vi "Henries Converter.vi"(1 "L in":dbl, 2 "L Units":enum16{"H", "mH", "µH", "nH", "pH"}(ring)) -> (0 "L out":dbl)   [LabVIEW 2013]
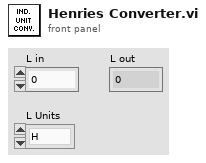
[diagram p1: front panel]
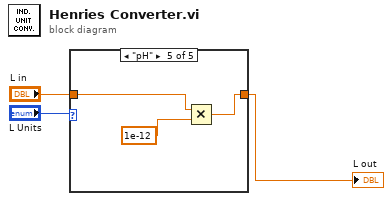
[diagram p0: block diagram]
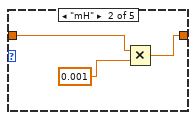
[diagram p3: hidden frame]
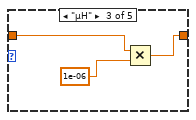
[diagram p4: hidden frame]
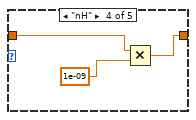
[diagram p5: hidden frame]
diagram:
  n1 = case shown="\"pH\"" "L Units" {
    tunnel: "L in" -> [w4 w7 w10 w13 w16]
    tunnel: [w4 w6 w9 w12 w15] -> w3
    frame "H", Default {
    }
    frame "mH" {
      n2 = Multiply(x=w7, y=0.001) -> (x*y=w6:dbl)
    }
    frame "µH" {
      n3 = Multiply(x=w10, y=1e-06) -> (x*y=w9:dbl)
    }
    frame "nH" {
      n4 = Multiply(x=w13, y=1e-09) -> (x*y=w12:dbl)
    }
    frame "pH" {
      n5 = Multiply(x=w16, y=1e-12) -> (x*y=w15:dbl)
    }
  }
  "L out" <- w3
